vi "AlwaysPID.vi"() -> ()   [LabVIEW 2012]
uses:
  State_Machine_Enum.ctl
  <vilib>/Rock Robotics/WPI/RobotDrive/WPI_RobotDriveGetSetRefNum.vi
  Robot Global Data.vi
  <vilib>/addons/control/pid/pid.llb/PID (DBL).vi
  <vilib>/addons/control/pid/NI_PID_pid.lvlib
panel:
  in  "Output Range":cluster{"Output Max":dbl, "Output Min":dbl}={"Output Max"=1.0, "Output Min"=-1.0} {"Output Min" min=-1.1 max=0.1 step=0.1; "Output Max" min=-0.1 max=1.1 step=0.1}
  in  "PID Gains":T1={"Proportional Gain (Kc)"=2.4, "Integral Time (Ki, sec)"=4.8, "Derivative Time (Kd, sec)"=0.3} {"Derivative Time (Kd, sec)" min=-0.01 max=1.01 step=0.01; "Integral Time (Ki, sec)" min=-0.01 max=10.0 step=0.01; "Proportional Gain (Kc)" min=-0.1 max=5.1 step=0.01}
  # "Defaults: \nKc: 2.4\nKi:  4.8\nKd: 0.3"
  # "Defaults: \nMax 0\nMin -1"
  # "HOW TO CALCULATE PID VALUES:\n1) Find time to accelerate to max speed. (In this case, \n     .5 sec.) This is T.\n2) Assume delay between start / max acceleration \n     is 1/2 of value in step 1. This is L.\n3) Calculate PID values:\n     P: 1.2 (T/L)\n     I: .6(T/L^2)\n     D: .6T\n(This is the dumbed-down version.)"
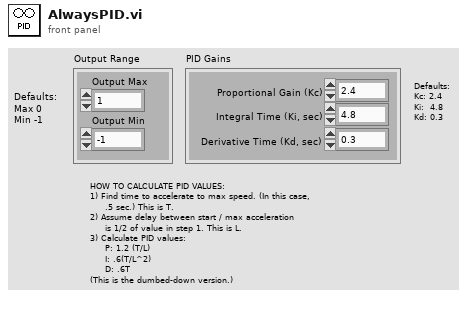
[diagram p1: front panel]
types:
  T1 = cluster{"Proportional Gain (Kc)":dbl, "Integral Time (Ki, sec)":dbl, "Derivative Time (Kd, sec)":dbl}
  T2 = typedef "State_Machine_Enum.ctl" = enum16{"Init", "Idle", "Start", "Do", "Stop"}
  T3 = typedef "WPI_RobotDriveDevRef.ctl" = cluster{"DevStatus":errorcluster, "Motors[]":T4[], "Square Inputs":bool, "Max Output":dbl, "Isochronous":bool}
  T4 = typedef "WPI_MotorControlDeviceRef.ctl" = cluster{"DeviceStatus":errorcluster, "Type":enum16{"PWM", "CAN"}, "PWM":cluster{"Digital Module":T5, "PWM Channel":T6, "DeadBand":T7}, "CAN":cluster{"Device Number":u8, "Control Mode":T8, "Semaphore":T9, "Max Vout":dbl}, "Invert":bool, "TransformRef":T10, "InvTransformRef":T10}
  T5 = typedef "FPGA_TypedefDigitalModule.ctl" = enum16{"Digital Module 1", "Digital Module 2"}
  T6 = typedef "FPGA_DIOPWMChannel.ctl" = enum8{"PWM 1", "PWM 2", "PWM 3", "PWM 4", "PWM 5", "PWM 6", "PWM 7", "PWM 8", "PWM 9", "PWM 10", "Invalid"}
  T7 = typedef "WPI_PWMDeadband.ctl" = cluster{"Name":string, "maxPositivePwm":i32, "minPositivePwm":i32, "centerPwm":i32, "maxNegativePwm":i32, "minNegativePwm":i32, "angularRange":u16}
  T8 = typedef "WPI_CANJaguar_ControlMode.ctl" = enum8{"Percent VBus", "Current", "Speed", "Position", "Voltage"}
  T9 = typedef "Semaphore RefNum" = refnum<k1>
  T10 = typedef "WPI_PWMTransform_ConPane.ctl" = refnum<vi>
  T11 = typedef "WPI_EncoderDevRef.ctl" = cluster{"DevStatus":errorcluster, "EncoderIndex":T12, "CounterIndex":T13, "DistancePerCount":dbl, "Decoding Type":T14}
  T12 = typedef "FPGA_EncoderIdx.ctl" = enum8{"Enc 0", "Enc 1", "Enc 2", "Enc 3", "Invalid"}
  T13 = typedef "FPGA_CounterCtrSystemIndex.ctl" = enum8{"Ctr 0", "Ctr 1", "Ctr 2", "Ctr 3", "Ctr 4", "Ctr 5", "Ctr 6", "Ctr 7", "Invalid"}
  T14 = typedef "WPI_EncoderType.ctl" = enum16{"1x", "2x", "4x"}
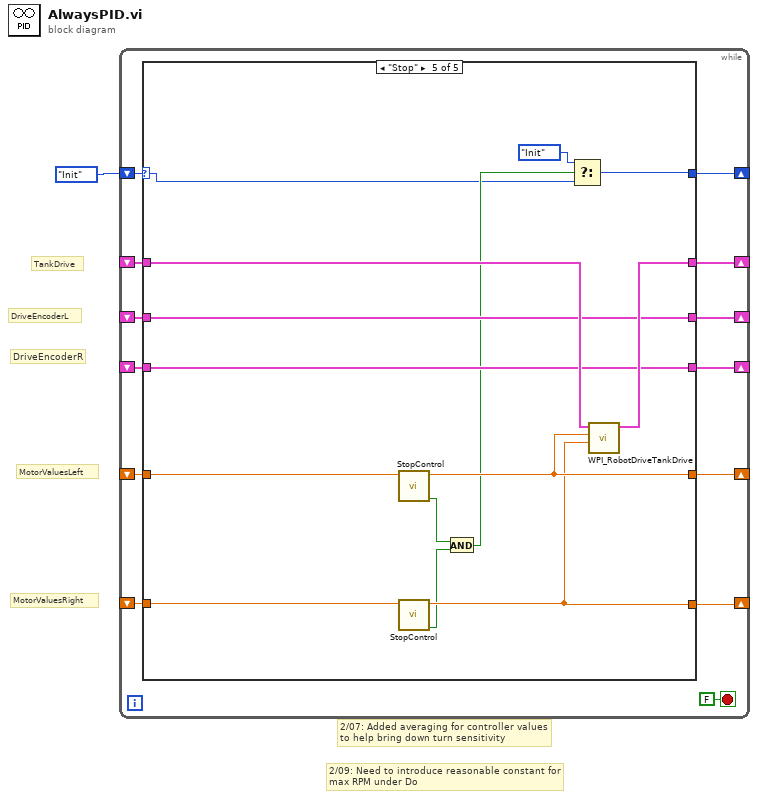
[diagram p0: block diagram]
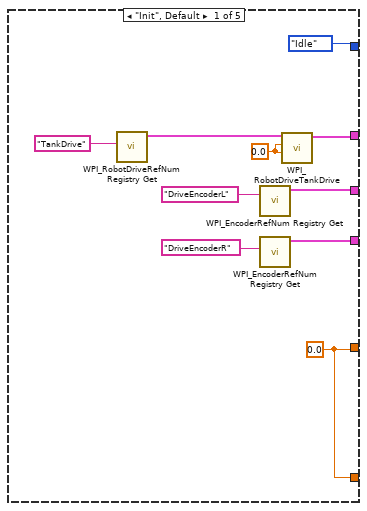
[diagram p2: hidden frame]
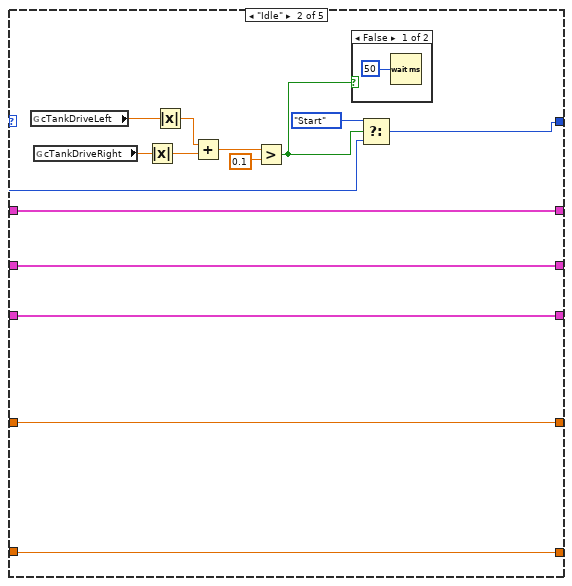
[diagram p3: hidden frame]
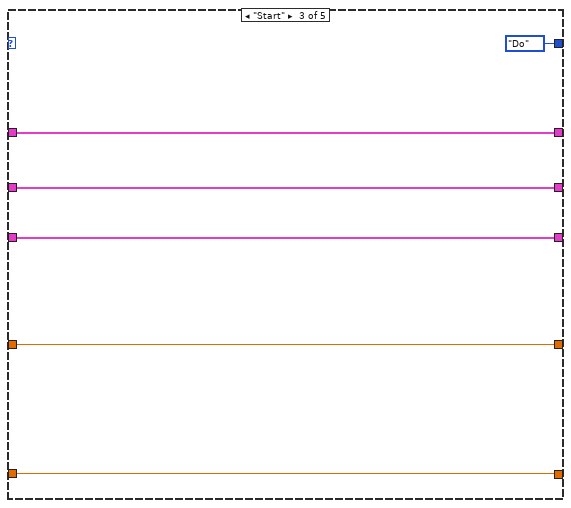
[diagram p5: hidden frame]
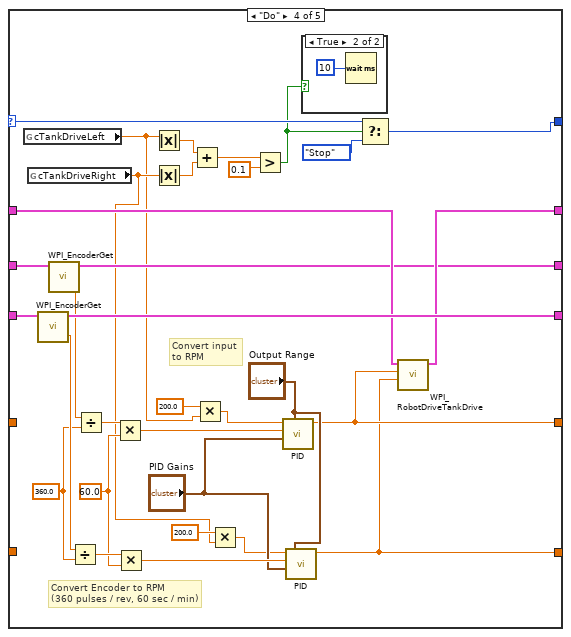
[diagram p6: hidden frame]
diagram:
  # "MotorValuesRight"
  # "MotorValuesLeft"
  # "2/09: Need to introduce reasonable constant for\nmax RPM under Do"
  # "TankDrive"
  # "DriveEncoderR"
  # "DriveEncoderL"
  # "2/07: Added averaging for controller values\nto help bring down turn sensitivity"
  n1 = while {
    shift-right: [w12] -> _
    shift-left: State_Machine_Enum."Init" ("State") -> [w13]
    shift-right: [w11] -> _
    shift-left: _ -> [w10]
    shift-right: [w8] -> _
    shift-left: _ -> [w7]
    shift-right: [w9] -> _
    shift-left: _ -> [w6]
    shift-right: [w4] -> _
    shift-left: _ -> [w2]
    shift-right: [w5] -> _
    shift-left: _ -> [w3]
    stop <- FALSE stop-if-true
    n2 = case shown="\"Stop\"" w13 {
      selector: w13 -> [_ w34 _ w74 w81]
      tunnel: [State_Machine_Enum."Idle" ("State") w33 State_Machine_Enum."Do" ("State") w73 w80] -> w12
      tunnel: [w16 w27 w46 w57 w93] -> w11
      tunnel: w10 -> [_ w27 w46 w58 w92]
      tunnel: [w20 w29 w44 w56 w91] -> w9
      tunnel: [w19 w28 w43 w68 w90] -> w8
      tunnel: w7 -> [_ w28 w43 w70 w90]
      tunnel: w6 -> [_ w29 w44 w69 w91]
      tunnel: [w15 w26 w42 w48 w88] -> w5
      tunnel: [w15 w25 w41 w47 w87] -> w4
      tunnel: w3 -> [_ w26 w42 _ w89]
      tunnel: w2 -> [_ w25 w41 _ w86]
      frame "Init", Default {
        w15 = 0.0
        w18 = 0.0 ("Left axis value")
        n3 = call <vilib>:"WPI_RobotDriveRefNum Registry Get.vi"("refnum name"="TankDrive") -> ("RobotDriveDevRef"=w17:T3)  [unwired: 9 in, 1 out]
        n4 = call <vilib>:"WPI_EncoderRefNum Registry Get.vi"("refnum name"="DriveEncoderL") -> ("EncoderDevRef"=w20:T11)  [unwired: 9 in, 1 out]
        n5 = call <vilib>:"WPI_EncoderRefNum Registry Get.vi"("refnum name"="DriveEncoderR") -> ("EncoderDevRef"=w19:T11)  [unwired: 9 in, 1 out]
        n6 = call <vilib>:"WPI_RobotDriveTankDrive.vi"("Right axis value"=w18, "Left axis value"=w18, "RobotDriveDevRef"=w17) -> ("RobotDriveDevRef"=w16:T3)  [unwired: 6 in, 2 out]
      }
      frame "Idle" {
        n7 = global read "Robot Global Data.vi" "cTankDriveLeft"() -> (w32:dbl)
        n8 = global read "Robot Global Data.vi" "cTankDriveRight"() -> (w31:dbl)
        n9 = Absolute Value(x=w31) -> (abs(x)=w38:dbl)
        n10 = Absolute Value(x=w32) -> (abs(x)=w39:dbl)
        n11 = Add(x=w39, y=w38) -> (x+y=w37:dbl)
        n12 = Greater?(x=w37, y=0.1) -> (0:w35:bool)
        n13 = case shown="False" w35 {
          frame False {
            n14 = Wait (ms)(milliseconds to wait=u32 50) -> ()  [unwired: 1 out]
          }
          frame True {
          }
        }
        n15 = Select(t=State_Machine_Enum."Start" ("State"), s=w35, f=w34) -> (s? t:f=w33:T2)
      }
      frame "Start" {
      }
      frame "Do" {
        w55 = 60.0
        w65 = 360.0
        # "Convert input \nto RPM"
        # "Convert Encoder to RPM\n(360 pulses / rev, 60 sec / min)"
        n16 = global read "Robot Global Data.vi" "cTankDriveLeft"() -> (w49:dbl)
        n17 = global read "Robot Global Data.vi" "cTankDriveRight"() -> (w53:dbl)
        n18 = call <vilib>:"WPI_EncoderGet.vi"("EncoderDevRef"=w70) -> ("EncoderDevRef"=w68:T11, "Rate"=w67:dbl)  [unwired: 5 in, 4 out]
        n19 = call <vilib>:"WPI_EncoderGet.vi"("EncoderDevRef"=w69) -> ("EncoderDevRef"=w56:T11, "Rate"=w66:dbl)  [unwired: 5 in, 4 out]
        n20 = Divide(x=w67, y=w65) -> (x/y=w63:dbl)
        n21 = Divide(x=w66, y=w65) -> (x/y=w64:dbl)
        n22 = Multiply(x=w64, y=w55) -> (x*y=w62:dbl)
        n23 = Multiply(x=w63, y=w55) -> (x*y=w61:dbl)
        n24 = Absolute Value(x=w49) -> (abs(x)=w78:dbl)
        n25 = Absolute Value(x=w53) -> (abs(x)=w77:dbl)
        n26 = Add(x=w78, y=w77) -> (x+y=w75:dbl)
        n27 = Multiply(x=200.0, y=w49) -> (x*y=w51:dbl)
        n28 = Multiply(x=200.0, y=w53) -> (x*y=w52:dbl)
        n29 = Greater?(x=w75, y=0.1) -> (0:w72:bool)
        n30 = call-poly <vilib>:"PID.vi"("output range"="Output Range", "PID gains"="PID Gains", "process variable"=w62, "setpoint"=w51) -> ("output"=w48:dbl)  [unwired: 6 in, 1 out]
        n31 = call-poly <vilib>:"PID.vi"("output range"="Output Range", "PID gains"="PID Gains", "process variable"=w61, "setpoint"=w52) -> ("output"=w47:dbl)  [unwired: 6 in, 1 out]
        n32 = case shown="True" w72 {
          frame False {
          }
          frame True {
            n33 = Wait (ms)(milliseconds to wait=u32 10) -> ()  [unwired: 1 out]
          }
        }
        n34 = Select(t=w74, s=w72, f=State_Machine_Enum."Stop" ("State")) -> (s? t:f=w73:T2)
        n35 = call <vilib>:"WPI_RobotDriveTankDrive.vi"("Right axis value"=w47, "Left axis value"=w48, "RobotDriveDevRef"=w58) -> ("RobotDriveDevRef"=w57:T3)  [unwired: 6 in, 2 out]
      }
      frame "Stop" {
        n36 = call "StopControl.vi"("Motor Value"=w89) -> ("Done Stopping"=w85:bool, "New Motor Value"=w88:dbl)  [unwired: 9 in]
        n37 = call "StopControl.vi"("Motor Value"=w86) -> ("Done Stopping"=w84:bool, "New Motor Value"=w87:dbl)  [unwired: 9 in]
        n38 = And(x=w85, y=w84) -> (x .and. y?=w83:bool)
        n39 = Select(t=State_Machine_Enum."Init" ("State"), s=w83, f=w81) -> (s? t:f=w80:T2)
        n40 = call <vilib>:"WPI_RobotDriveTankDrive.vi"("Right axis value"=w87, "Left axis value"=w88, "RobotDriveDevRef"=w92) -> ("RobotDriveDevRef"=w93:T3)  [unwired: 6 in, 2 out]
      }
    }
  }
